vi "Timer Update.vi"(8 "error in (no error)":errorcluster, 10 "Timeout Value":i32=1000, 11 "Timing Engine in":refnum<class "Timing Engine.lvclass">) -> (0 "error out":errorcluster, 3 "Timing Engine out":refnum<class "Timing Engine.lvclass">)   [LabVIEW 2016, in "Assert API Components.lvlib" / "Assert Display.lvlib" / "Timing Engine.lvlib" / "Timing Engine.lvclass"]
uses:
  Timing Engine.lvclass
  Timing Engine.lvclass/Timing Engine.ctl
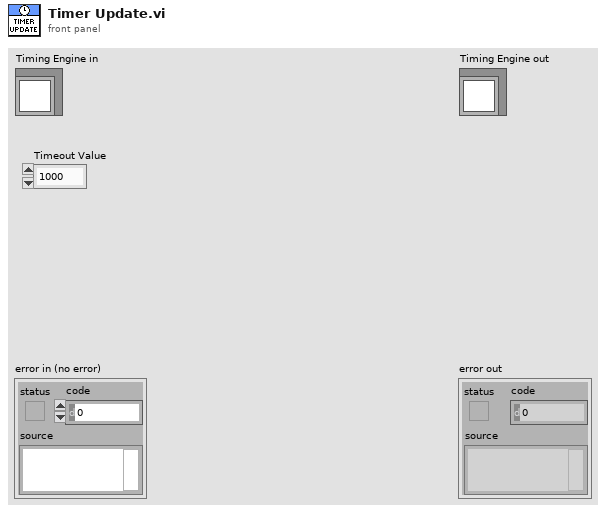
[diagram p1: front panel]
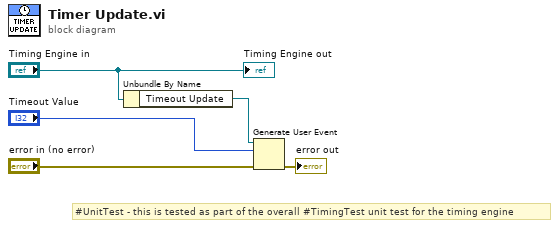
[diagram p0: block diagram]
diagram:
  # "#UnitTest - this is tested as part of the overall #TimingTest unit test for the timing engine"
  n1 = Unbundle By Name("Timing Engine in") -> ("Timeout Update"=w2:refnum<user-event>)
  n2 = Generate User Event(user event=w2, event data cluster="Timeout Value", error in="error in (no error)") -> (error out=→"error out":errorcluster)  [unwired: 1 in, 1 out]
  "Timing Engine out" <- "Timing Engine in"
